vi "adjustSetpoint(SubVI).vi"(5 "Current":sgl format="%#_6p", 7 "Bias (V)":sgl format="%_5p", 8 "error in (no error)":errorcluster, 9 "milliseconds to wait":u32, 10 "tipLift":dbl, 11 "Application in":refnum<vi>) -> (0 "error out":errorcluster, 3 "Application out":refnum<vi>)   [LabVIEW 2014]
uses:
  <userlib>/Nanonis Prog Interface V5/Nanonis Prog Interface.lvlib
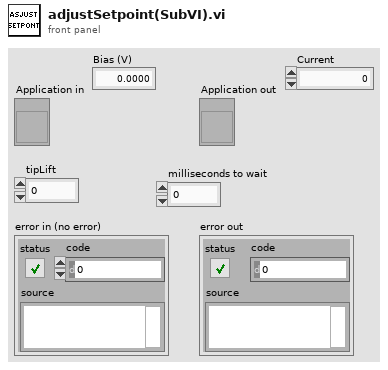
[diagram p1: front panel]
types:
  T1 = cluster{"X (m)":sgl, "Y (m)":sgl, "Text":string, "Color":u32, "Visible":bool}[]
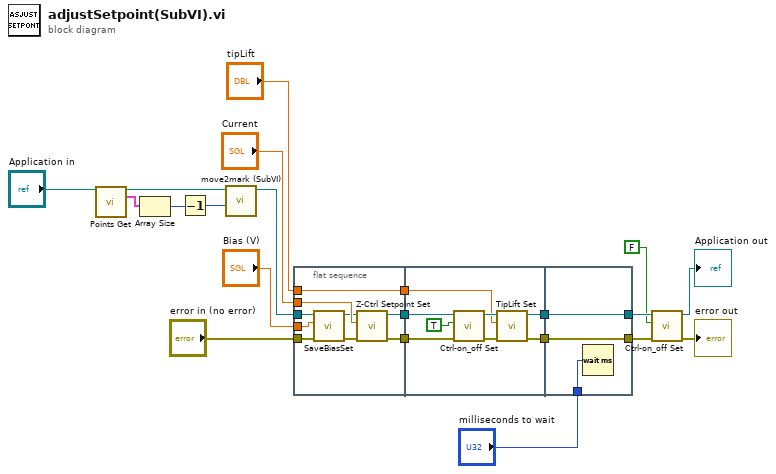
[diagram p0: block diagram]
diagram:
  n1 = call <userlib>:"Points Get.vi"("Application ref in"="Application in") -> ("Application ref out"=w6:refnum<vi>, "Points"=w10:T1)  [unwired: 12 in, 1 out]
  n2 = Array Size(array=w10) -> (size(s)=w9:i32)
  n3 = Decrement(x=w9) -> (x-1=w8:i32)
  n4 = call "move2mark (SubVI).vi"("index"=w8, "Application in"=w6) -> ("Application out"=w18:refnum<vi>)  [unwired: 9 in]
  n5 = flat-sequence {
    tunnel: "tipLift" -> [w30]
    tunnel: w18 -> [w26]
    tunnel: "error in (no error)" -> [w25]
    tunnel: [w28] -> w5
    tunnel: [w29] -> w4
    tunnel: [w30] -> w3
    tunnel: "Bias (V)" -> [w22]
    tunnel: "Current" -> [w27]
    tunnel: [w34] -> w14
    tunnel: [w33] -> w13
    tunnel: w5 -> [w38]
    tunnel: w4 -> [w35]
    tunnel: w3 -> [w32]
    tunnel: [w40] -> w16
    tunnel: [w41] -> w17
    tunnel: w14 -> [w41]
    tunnel: w13 -> [w40]
    tunnel: "milliseconds to wait" -> [w39]
    frame #0 {
      n6 = call "SaveBiasSet.vi"("Application ref in"=w26, "Bias (V)"=w22, "error in (no error)"=w25) -> ("Application ref out"=w24:refnum<vi>, "Error out"=w23:errorcluster)  [unwired: 6 in]
      n7 = call <userlib>:"Z-Ctrl Setpoint Set.vi"("error in (no error)"=w23, "Z Controller setpoint"=w27, "Application ref in"=w24) -> ("error out"=w28:errorcluster, "Application ref out"=w29:refnum<vi>)  [unwired: 7 in]
    }
    frame #1 {
      n8 = call <userlib>:"Ctrl-on_off Set.vi"("error in (no error)"=w38, "Z Controller ON/OFF"=TRUE, "Application ref in"=w35) -> ("error out"=w37:errorcluster, "Application ref out"=w36:refnum<vi>)  [unwired: 7 in]
      n9 = call <userlib>:"TipLift Set.vi"("error in (no error)"=w37, "TipLift (m)"=w32, "Application ref in"=w36) -> ("error out"=w34:errorcluster, "Application ref out"=w33:refnum<vi>)  [unwired: 7 in]
    }
    frame #2 {
      n10 = Wait (ms)(milliseconds to wait=w39) -> ()  [unwired: 1 out]
    }
  }
  n11 = call <userlib>:"Ctrl-on_off Set.vi"("error in (no error)"=w17, "Z Controller ON/OFF"=FALSE, "Application ref in"=w16) -> ("error out"=→"error out":errorcluster, "Application ref out"=→"Application out":refnum<vi>)  [unwired: 7 in]
